vi "Configure Modulation (PSK).vi"(0 "VISA resource name":refnum<visa-resource-name>, 1 "Enable PSK Modulation (T: Enable)":bool=TRUE, 3 "Peak Deviation Unit (0: Radian)":u16(ring) items=["Radians", "Degrees"], 5 "Channel (1: Channel 1)":u16(ring)=1 items=["Channel 1"=1, "Channel 2"=2], 7 "PSK Modulation Source (0: Internal)":u16(ring) items=["Internal", "External"], 9 "Peak Deviation (0)":dbl format="%.2f", 11 "error in (no error)":errorcluster, 12 "Internal Rate (100.00 Hz)":dbl=100.0 format="%.2f") -> (4 "VISA resource name out":refnum<visa-resource-name>, 15 "error out":errorcluster)   [LabVIEW 2016, in "Tektronix AFG 1000 Series.lvlib"]
doc: "Configures and enables Amplitude-Shift Keying (PSK) modulation.\n\n<b>Note:</b>\nThis VI is not supported for AFG1022."
uses:
  Tektronix AFG 1000 Series.lvlib
panel:
  # "Internal PSK Settings"
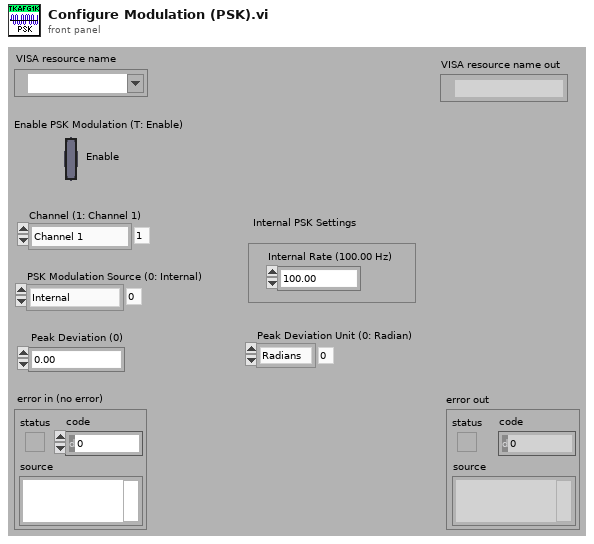
[diagram p1: front panel]
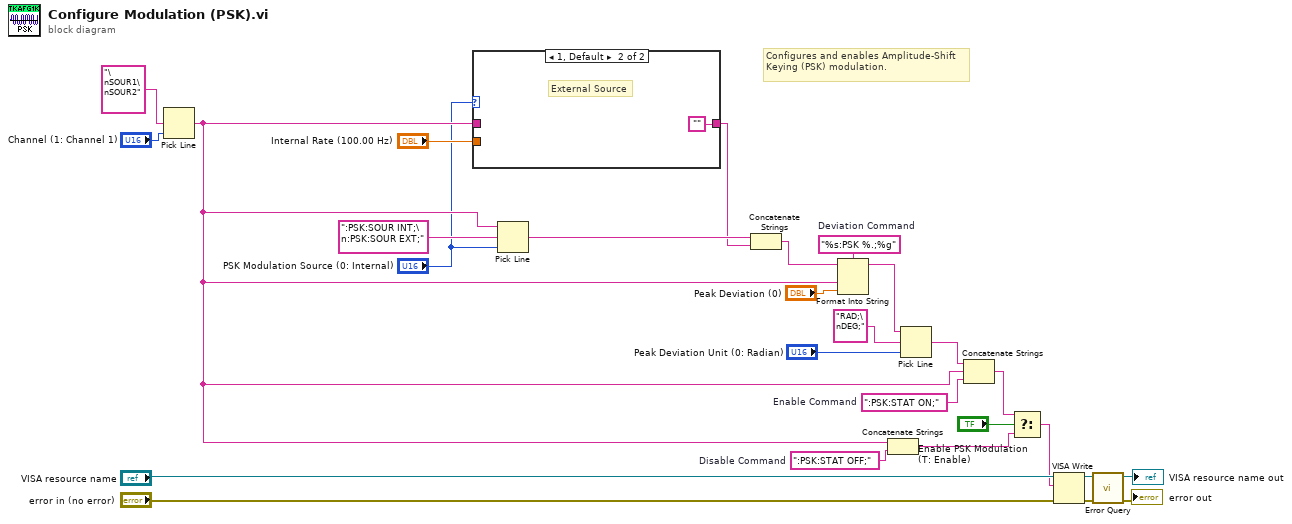
[diagram p0: block diagram]
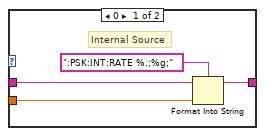
[diagram p2: hidden frame]
diagram:
  w21 = "%s:PSK %.;%g"  # Deviation Command
  w7 = ":PSK:STAT ON;"  # Enable Command
  w14 = ":PSK:STAT OFF;"  # Disable Command
  # "Configures and enables Amplitude-Shift Keying (PSK) modulation."
  n1 = Pick Line(multi-line string="\nSOUR1\nSOUR2" ("string (\"\")"), line index="Channel (1: Channel 1)") -> (output string=w6:string)  [unwired: 1 in]
  n2 = case shown="1, Default" "PSK Modulation Source (0: Internal)" {
    tunnel: [w30 ""] -> w11
    tunnel: w6 -> [w29 _]
    tunnel: "Internal Rate (100.00 Hz)" -> [w28 _]
    frame 0 {
      # "Internal Source"
      n3 = Format Into String(format string=":PSK:INT:RATE %.;%g;" ("initial string"), initial string=w29, w28) -> (resulting string=w30:string)  [unwired: 1 in, 1 out]
    }
    frame 1, Default {
      # "External Source"
    }
  }
  n4 = Pick Line(string ("")=w6, multi-line string=":PSK:SOUR INT;\n:PSK:SOUR EXT;" ("string (\"\")"), line index="PSK Modulation Source (0: Internal)") -> (output string=w12:string)
  n5 = Concatenate Strings(w12, w11) -> (w10:string)
  n6 = Format Into String(format string=w21, initial string=w10, w6, "Peak Deviation (0)") -> (resulting string=w2:string)  [unwired: 1 in, 1 out]
  n7 = Concatenate Strings(w6, w14) -> (w13:string)
  n8 = Pick Line(string ("")=w2, multi-line string="RAD;\nDEG;", line index="Peak Deviation Unit (0: Radian)") -> (output string=w1:string)
  n9 = Concatenate Strings(w1, w6, w7) -> (w15:string)
  n10 = Select(t=w15, s="Enable PSK Modulation (T: Enable)", f=w13) -> (s? t:f=w16:string)
  n11 = VISA Write(VISA resource name="VISA resource name", write buffer=w16, error in (no error)="error in (no error)") -> (VISA resource name out=w26:refnum<visa-resource-name>, error out=w25:errorcluster)  [unwired: 1 out]
  n12 = call "Error Query.vi"("error in (no error)"=w25, "VISA resource name"=w26) -> ("error out"=→"error out":errorcluster, "VISA resource name out"=→"VISA resource name out":refnum<visa-resource-name>)  [unwired: 6 in, 2 out]
